vi "SEA_TRANSPARENCY_MOTOR_CURRENT_CTL_TESTING.vi"() -> ()   [LabVIEW 2019]
uses:
  <vilib>/Platform/TimedLoop/XDataNode/timing_clust.ctl
  <vilib>/Platform/TimedLoop/XDataNode/nitl_modes.ctl
  <vilib>/Platform/TimedLoop/XDataNode/wakeup.ctl
  <vilib>/FPGAPlugInAG/sbRIO-9627/niLvFpga_Open_sbRIO-9627.vi
  <vilib>/rvi/interface/common/dynamic/niFpgaDynamicAddResources.vi
  <vilib>/Utility/error.llb/Error Cluster From Error Code.vi
  <vilib>/rvi/errors/niLvFpgaAdjustHostInterfaceError.vi
  <vilib>/FPGAPlugInAG/Dynamic/niLvFpga_Close_Dynamic.vi
  <vilib>/rvi/interface/nirviOpenFPGA/nirviOpenFPGA.xnode
  FPGA Bitfiles/seafinalexperime_FPGATarget_SEALOWERLEVELPIC_AplcQzvwIw0.lvbitx
  SEA_LOWER_LEVEL_PI_CONTROL.vi
  <vilib>/platform/TimedLoop/XDataNode/XDataNode.xnode
  <vilib>/rvi/interface/nirviReadWriteControl/nirviReadWriteControl.xnode
  <vilib>/rvi/interface/nirviCloseFPGA/nirviCloseFPGA.xnode
  <vilib>/Platform/TimedLoop/XDataNode/XDNodeRunTimeDep.lvlib
  NiFpgaLv.dll
  <vilib>/rvi/interface/Simulation/niFpgaSimulationCallBeginRW.vi
panel:
  out "Motor position":T1(graph)
  out "Transparent motor current":T2(graph)
  out "Finished late?":u32
  in  "Amplitude":sgl
  in  "frequency":sgl
  out "transparency Motor direction":bool
  out "transparency control_ip":sgl
  in  "transparency motor Upper bound":sgl
  in  "transparency motor Lower bound":sgl
  in  "transparency motor Ki current control":sgl
  in  "transparency motor Kp current control":sgl
  in  "transparency Current Offset":sgl
  in  "Position Reset transparency side":bool
  in  "Position Reset joint side":bool
  out "filtered current":sgl
  out "Motor direction":bool
  out "control_ip":sgl
  in  "Lower bound":sgl
  in  "Upper bound":sgl
  in  "Ki current control":sgl
  in  "Kp current control":sgl
  in  "Current Offset":sgl
  in  "stop":bool
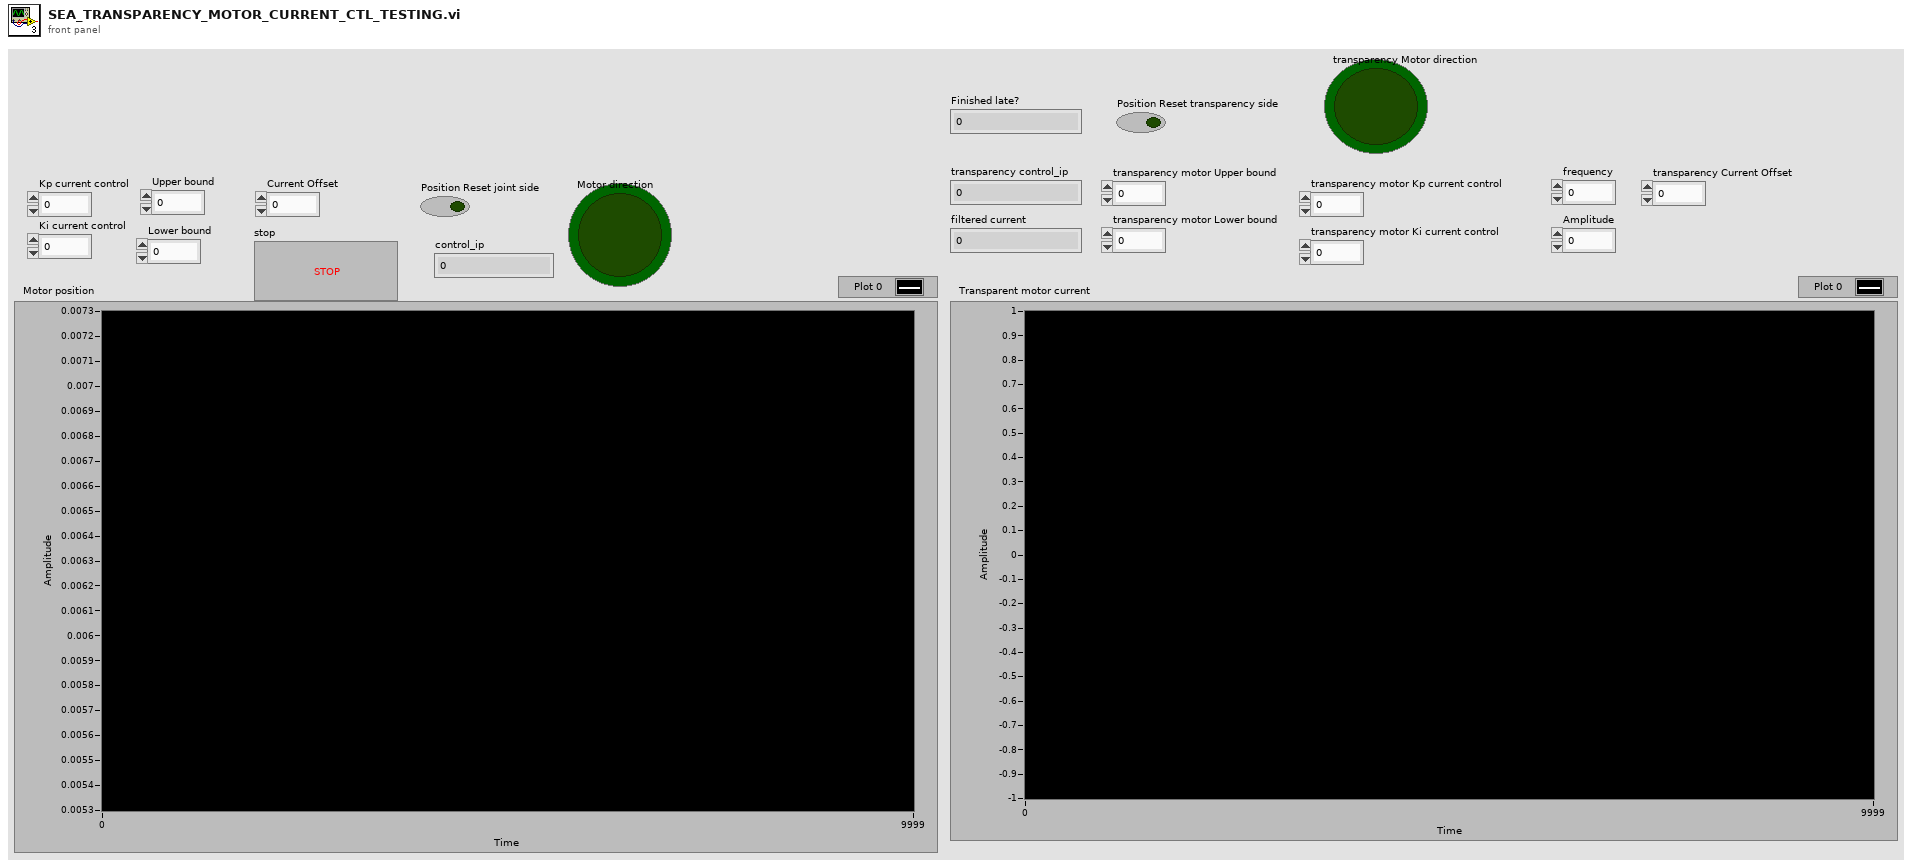
[diagram p1: front panel]
types:
  T1 = cluster{"Position(Radians) transparency motor side":sgl, "Position(Radians) joint side":sgl}
  T2 = cluster{sgl, "transparency filtered current":sgl}
  T3 = typedef "XDNodeRunTimeDep.lvlib/timing_clust.ctl" = cluster{"Expected End [f-1]":u64, "Actual End [f-1]":u64, "Finished Late? [f-1]":bool, "Expected End [i-1]":u64, "Actual End [i-1]":u64, "Finished Late? [i-1]":bool, "Expected Start [i]":u64, "Actual Start [i]":u64, "Expected Start [f]":u64, "Actual Start [f]":u64, "Source Name":string, "Structure Name":string, "Period":i64, "Deadline":i64, "Offset":i64, "Start":i64, "Priority":i32, "Timeout":i32, "Mode":T4, "Wakeup Reason":T5, "Error":errorcluster, "Source Type":string, "Secondary Source Type":string, "Global End Time":u64, "Global Start Time":u64, "Frame Duration":u64, "Iteration Duration":u64, "Assigned CPU":i32, "I/O Scan Engine Mode":u32}
  T4 = typedef "XDNodeRunTimeDep.lvlib/nitl_modes.ctl" = enum32{"No Change", "Process missed periods, maintain original phase", "Discard missed periods, maintain original phase", "Process missed periods, ignore original phase", "Discard missed periods, ignore original phase"}
  T5 = typedef "XDNodeRunTimeDep.lvlib/wakeup.ctl" = enum32{"Normal", "Aborted", "Asynchronous wakeup", "Timing source error", "Timed loop error", "Timeout"}
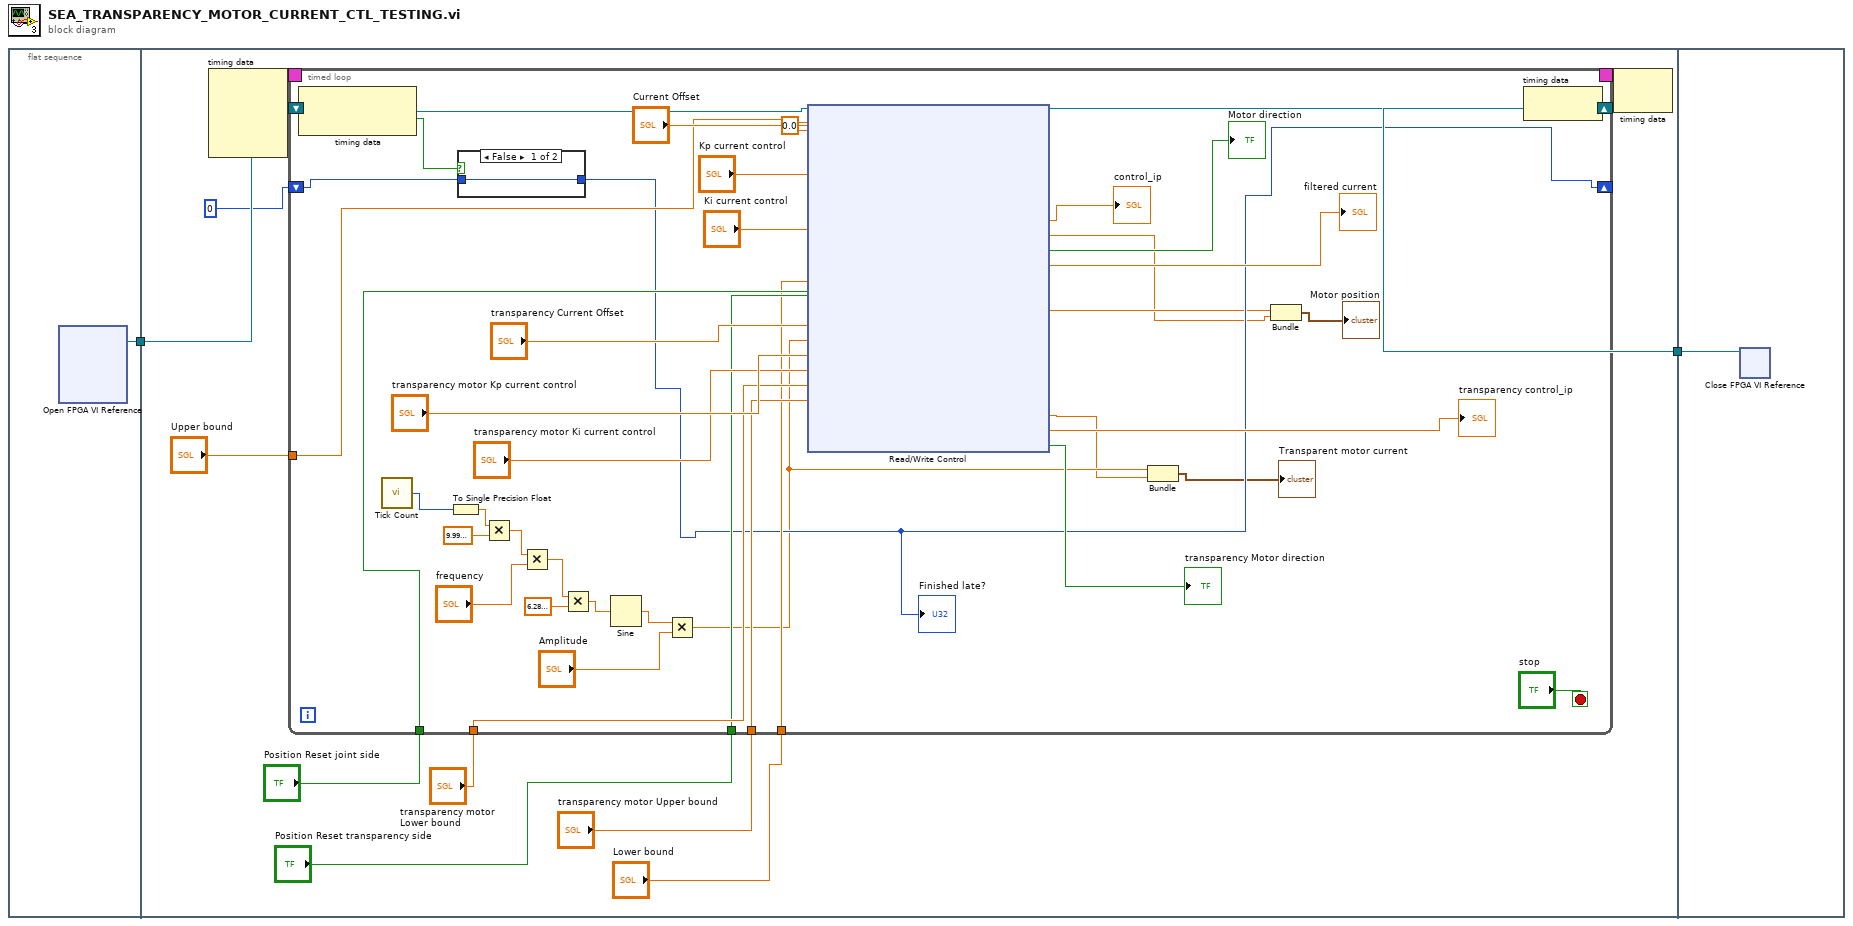
[diagram p0: block diagram]
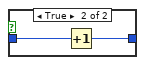
[diagram p2: hidden frame]
diagram:
  n1 = flat-sequence {
    tunnel: [w3] -> w2
    tunnel: w2 -> [w14]
    tunnel: [w13] -> w1
    tunnel: w1 -> [w63]
    frame #0 {
      n2 = xnode "Open FPGA VI Reference"() -> ("FPGA VI Reference Out"=w3:refnum<k20>)  [unwired: 2 in, 1 out]
    }
    frame #1 {
      n3 = node-c288() -> (w12:T3)  [unwired: 4 in]
      n4 = timed-loop {
        timing: w12 -> [_]
        timing-out: [_] -> w11
        shift-right: [w53] -> w13
        shift-left: w14 -> [w54]
        tunnel: "transparency motor Upper bound" -> [w40]
        tunnel: "transparency motor Lower bound" -> [w39]
        tunnel: "Position Reset transparency side" -> [w38]
        tunnel: "Position Reset joint side" -> [w37]
        tunnel: "Lower bound" -> [w36]
        tunnel: "Upper bound" -> [w35]
        shift-right: [w21] -> _
        shift-left: u32 0 -> [w22]
        stop <- "stop" stop-if-true
        n5 = node-c288() -> (w23:bool)  [unwired: 1 in, 1 out]
        n6 = call "Tick Count"() -> ("Tick Count(uSec)"=w24:u32)
        n7 = To Single Precision Float(number=w24) -> (single precision float=w34:sgl)
        n8 = case shown="False" w23 {
          tunnel: w22 -> [w55 w57]
          tunnel: [w55 w56] -> w21
          frame False {
          }
          frame True {
            n9 = Increment(x=w57) -> (x+1=w56:u32)
          }
        }
        "Finished late?" <- w21
        n10 = Multiply(x=w34, y=sgl 1e-06) -> (x*y=w32:sgl)
        n11 = Multiply(x=w32, y="frequency") -> (x*y=w30:sgl)
        n12 = Multiply(x=w30, y=sgl 6.28) -> (x*y=w28:sgl)
        n13 = Sine(x=w28) -> (sin(x)=w27:sgl)
        n14 = Multiply(x=w27, y="Amplitude") -> (x*y=w20:sgl)
        n15 = xnode "Read/Write Control"("FPGA VI Reference In"=w54, "Current Offset"="Current Offset", "Reference"=sgl 0.0, "Kp current control"="Kp current control", "Ki current control"="Ki current control", "Upper bound"=w35, "Lower bound"=w36, "Position Reset joint side"=w37, "Position Reset transparency side"=w38, "transparency Current Offset"="transparency Current Offset", "transparency reference"=w20, "transparency motor Kp current control"="transparency motor Kp current control", "transparency motor Ki current control"="transparency motor Ki current control", "transparency motor Lower bound"=w39, "transparency motor Upper bound"=w40) -> ("FPGA VI Reference Out"=w53:refnum<k20>, "control_ip"=→"control_ip":sgl, "Position(Radians) joint side"=w16:sgl, "Motor direction"=→"Motor direction":bool, "filtered current"=→"filtered current":sgl, "Position(Radians) transparency motor side"=w17:sgl, "transparency filtered current"=w19:sgl, "transparency control_ip"=→"transparency control_ip":sgl, "transparency Motor direction"=→"transparency Motor direction":bool)  [unwired: 1 in, 1 out]
        n16 = Bundle(w20, "transparency filtered current"=w19) -> (→"Transparent motor current":T2)  [unwired: 1 in]
        n17 = Bundle("Position(Radians) transparency motor side"=w17, "Position(Radians) joint side"=w16) -> (→"Motor position":T1)  [unwired: 1 in]
        n18 = node-c288() -> ()  [unwired: 1 in, 1 out]
      }
      n19 = node-c288(w11) -> ()  [unwired: 1 out]
    }
    frame #2 {
      n20 = xnode "Close FPGA VI Reference"("FPGA VI Reference In"=w63) -> ()  [unwired: 1 in, 1 out]
    }
  }
